vi "pixel2milimetr.vi"(0 "session in":refnum<k35>, 1 "module path":path, 5 "3*3 Transform Matrix":sgl[][](array[numeric]), 7 "factor":sgl, 9 "circle array":dbl[][](array[numeric]), 11 "Error in":errorcluster, 12 "function name":string) -> (4 "session out":refnum<k35>, 8 "calibrated circles":dbl[][](array[numeric]), 15 "Error out":errorcluster)   [LabVIEW 2019]
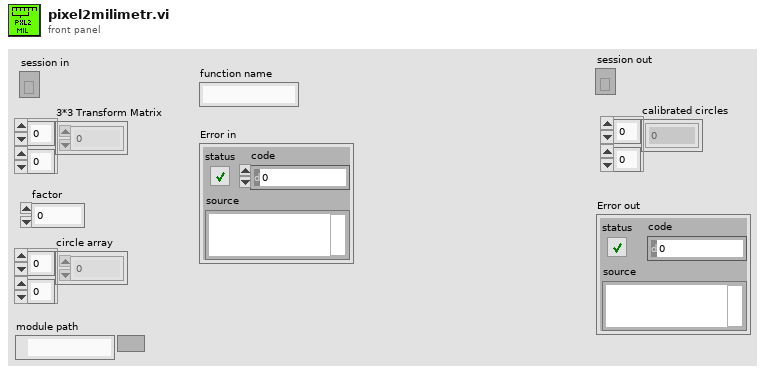
[diagram p1: front panel]
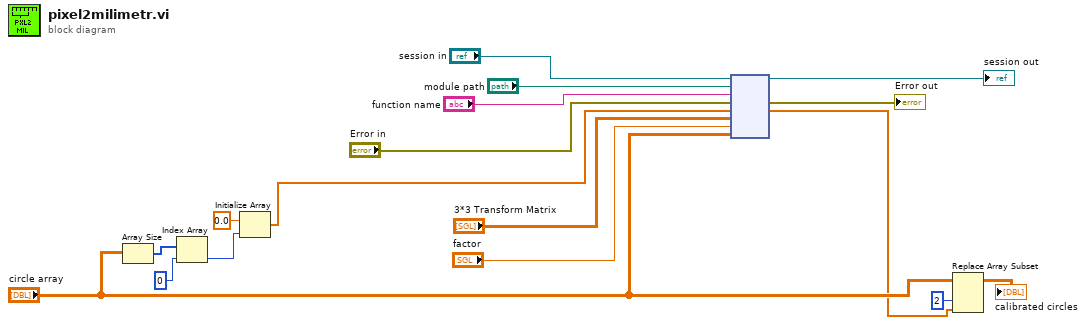
[diagram p0: block diagram]
diagram:
  n1 = Array Size(array="circle array") -> (size(s)=w9:i32[])
  n2 = Index Array(array=w9, index=0) -> (element=w6:i32)
  n3 = Initialize Array(sgl 0.0 ("element"), w6) -> (w5:sgl[])
  n4 = node("session in", "module path", "function name", "Error in", w5, "3*3 Transform Matrix", "factor", "circle array") -> (→"session out":refnum<k35>, →"Error out":errorcluster, w2:sgl[])  [unwired: 3 in, 2 out]
  n5 = Replace Array Subset(array="circle array", new element=w2, index (col)=2 ("disabled index (col)")) -> (→"calibrated circles":dbl[][])  [unwired: 1 in]
